vi "Configure Level Qualifier.vi"(6 "Condition (0: High)":i32(ring) items=["High", "Low", "Inside", "Outside"], 7 "Enable Level Qualifying (F: Disable)":bool, 8 "error in (no error)":errorcluster, 9 "Qualifier (1: Qualifier1)":i32(ring)=1 items=["Qualifier1"=1, "Qualifier2"=2, "Qualifier3"=3], 10 "Channel (1: Channel1)":i32(ring)=1 items=["Channel1"=1, "Channel2"=2, "Channel3"=3, "Channel4"=4], 11 "VISA resource name":refnum<visa-resource-name>) -> (0 "error out":errorcluster, 3 "VISA resource name out":refnum<visa-resource-name>)   [LabVIEW 2020, in "Agilent 90000 Series.lvlib"]
doc: "Configures the level qualifiers."
uses:
  Agilent 90000 Series.lvlib
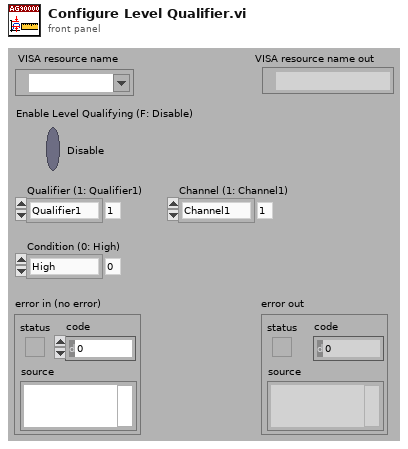
[diagram p1: front panel]
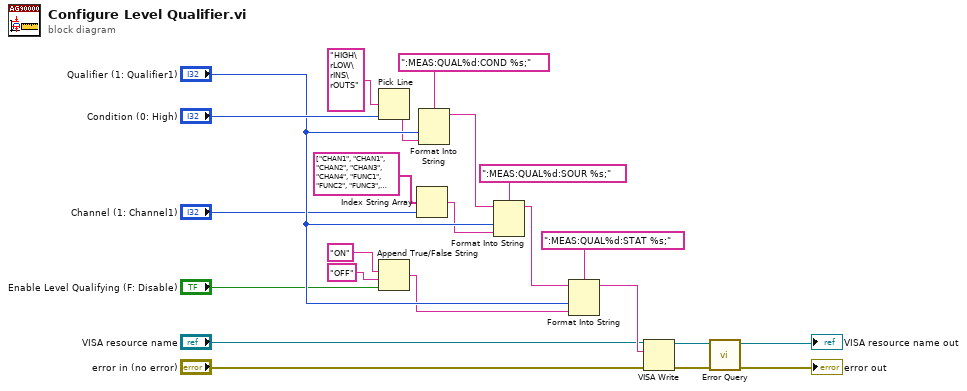
[diagram p0: block diagram]
diagram:
  n1 = Pick Line(multi-line string="HIGH\rLOW\rINS\rOUTS", line index="Condition (0: High)") -> (output string=w19:string)  [unwired: 1 out]
  n2 = Append True/False String(1:"Enable Level Qualifying (F: Disable)", 2:"OFF", 3:"ON") -> (0:w11:string)  [unwired: 1 out]
  n3 = Index String Array(1:"Channel (1: Channel1)", 2:string[] ["CHAN1", "CHAN1", "CHAN2", "CHAN3", "CHAN4", "FUNC1", "FUNC2", "FUNC3", "FUNC4", "WMEM1", "WMEM2", "WMEM3", "WMEM4"] ("subarray 2")) -> (0:w6:string)  [unwired: 1 in]
  n4 = Format Into String(format string=":MEAS:QUAL%d:COND %s;", "Qualifier (1: Qualifier1)", w19) -> (resulting string=w17:string)  [unwired: 2 in, 1 out]
  n5 = Format Into String(format string=":MEAS:QUAL%d:SOUR %s;", initial string=w17, "Qualifier (1: Qualifier1)", w6) -> (resulting string=w12:string)  [unwired: 1 in, 1 out]
  n6 = Format Into String(format string=":MEAS:QUAL%d:STAT %s;", initial string=w12, "Qualifier (1: Qualifier1)", w11) -> (resulting string=w10:string)  [unwired: 1 in, 1 out]
  n7 = VISA Write(VISA resource name="VISA resource name", write buffer=w10, error in (no error)="error in (no error)") -> (VISA resource name out=w5:refnum<visa-resource-name>, error out=w4:errorcluster)  [unwired: 1 out]
  n8 = call "Error Query.vi"("error in (no error)"=w4, "VISA resource name"=w5) -> ("error out"=→"error out":errorcluster, "VISA resource name out"=→"VISA resource name out":refnum<visa-resource-name>)  [unwired: 8 out]
